vi "20220114_03.vi"() -> ()   [LabVIEW 2019]
panel:
  in  "Stop":bool
  out "data":string
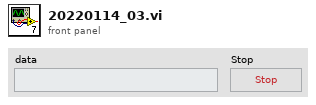
[diagram p1: front panel]
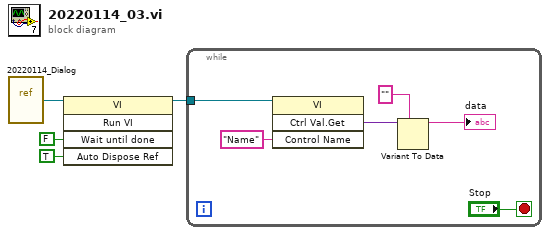
[diagram p0: block diagram]
diagram:
  n1 = vi-ref "20220114_Dialog.vi"() -> (w4:refnum<vi>)
  n2 = invoke class="VI" method="Run VI"(reference=w4, "Wait until done"=FALSE ("Wait Until Done"), "Auto Dispose Ref"=TRUE ("Auto Dispose Reference")) -> (reference out=w3:refnum<vi>)  [unwired: 2 in, 4 out]
  n3 = while {
    tunnel: w3 -> [w10]
    stop <- "Stop" stop-if-true
    n4 = invoke class="VI" method="Ctrl Val.Get"(reference=w10, "Control Name"="Name") -> ("Get Control Value Variant"=w9:variant)  [unwired: 2 in, 3 out]
    n5 = Variant To Data(type="", Variant=w9) -> (data=→"data":string)  [unwired: 1 in, 1 out]
  }
